vi "Do.vi"(8 "error in (no error)":errorcluster, 10 "Actor in":refnum<class "Actor.lvclass">, 11 "Analyse Board Msg":refnum<class "Analyse Board Msg.lvclass">) -> (0 "error out":errorcluster, 2 "Actor out":refnum<class "Actor.lvclass">)   [LabVIEW 2014, in "GoBang.lvlib" / "Analyse Board Msg.lvclass"]
doc: "This VI delivers the message to the actor by calling the appropriate method(s) on the actor."
uses:
  Analyse Board Msg.lvclass
  Server/CS++GoBangServer.lvclass
  CS++/Packages/CSPP_Core/Actors/CS++PVMonitor Messages/CS++PVUpdate Msg/CS++PVUpdate Msg.lvclass
  CS++/Packages/CSPP_Core/Classes/CS++ProcessVariables/ProcessVariable/PV.lvclass
  <vilib>/ActorFramework/Actor/Actor.lvclass
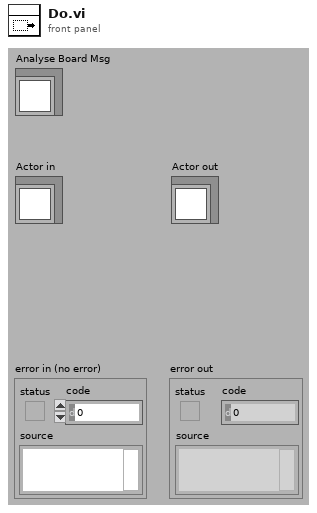
[diagram p1: front panel]
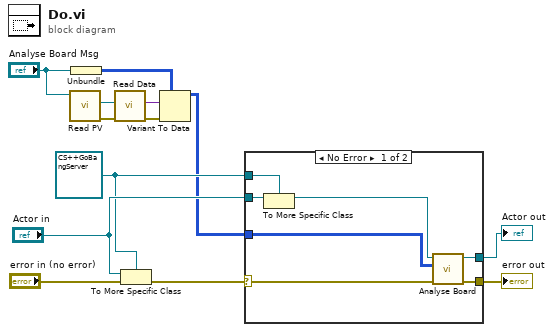
[diagram p0: block diagram]
diagram:
  w4 = refnum<class "CS++GoBangServer.lvclass"> refnum ("Actor in")
  n1 = call "Read PV.vi"("CS++PVUpdate Msg in"="Analyse Board Msg") -> ("error out"=w5:errorcluster, "PV"=w6:refnum<class "PV.lvclass">)  [unwired: 8 in, 1 out]
  n2 = Unbundle("Analyse Board Msg") -> (w2:u8[][])
  n3 = call "Read Data.vi"("error in (no error)"=w5, "PV in"=w6) -> ("error out"=w7:errorcluster, "Data"=w8:variant)  [unwired: 7 in, 1 out]
  n4 = To More Specific Class(target class=w4, reference="Actor in", error in="error in (no error)") -> (error out=w12:errorcluster)  [unwired: 1 out]
  n5 = Variant To Data(error in=w7, type=w2, Variant=w8) -> (data=w1:u8[][])  [unwired: 1 out]
  n6 = case shown="No Error" w12 {
    selector: w12 -> [w18 w22]
    tunnel: [w20 w22] -> w11
    tunnel: [w19 w21] -> w10
    tunnel: "Actor in" -> [w17 w21]
    tunnel: w4 -> [w16 _]
    tunnel: w1 -> [w14 _]
    frame No Error {
      n7 = To More Specific Class(target class=w16, reference=w17) -> (specific class reference=w15:refnum<class "CS++GoBangServer.lvclass">)  [unwired: 1 in, 1 out]
      n8 = call-dynamic "Analyse Board.vi"("error in (no error)"=w18, "GameBoard"=w14, "CS++GoBangServer in"=w15) -> ("error out"=w20:errorcluster, "CS++GoBangServer out"=w19:refnum<class "CS++GoBangServer.lvclass">)  [unwired: 7 in]
    }
    frame Error {
      # "If type check fails, pass the original object out again."
    }
  }
  "error out" <- w11
  "Actor out" <- w10
